vi "flipYZu32.vi"(10 "pointIn":cluster{"X":dbl, "Y":dbl, "Z":dbl}) -> (2 "pointOut":cluster{"X":dbl, "Y":dbl, "Z":dbl})   [LabVIEW 2015]
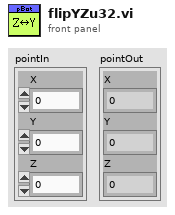
[diagram p1: front panel]
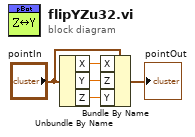
[diagram p0: block diagram]
diagram:
  n1 = Unbundle By Name("pointIn") -> ("X"=w4:dbl, "Y"=w3:dbl, "Z"=w2:dbl)
  n2 = Bundle By Name(cluster="pointIn", "X"=w4, "Z"=w3, "Y"=w2) -> (→"pointOut":cluster{"X":dbl, "Y":dbl, "Z":dbl})
